vi "e.gate HighSpeedPort Query - Base.vi"(0 "e.gate Configuration in":T1 {"StartTime" format="%#.10f"; "dActTimeToSecondFactor" format="%#.10f"; "StartTimeToDayFactor" format="%#_10f"}, 1 "Command":i32, 2 "OffsetWrite":i32, 3 "LengthWrite":i32, 4 "DataWrite":string="\u0000\t\f\u0000\u0000\u0000\u0000", 5 "OffsetRead":i32, 6 "LengthRead":i32, 7 "error in (no error)":errorcluster, 9 "TCP LengthReadt":i32, 11 "Timeout (1000)":i32) -> (20 "e.gate Configuration out":T1 {"StartTime" format="%#.10f"; "dActTimeToSecondFactor" format="%#.10f"; "StartTimeToDayFactor" format="%#_10f"}, 23 "Data (out binary)":u8[](array[numeric]), 24 "data out (string)":string, 27 "error out":errorcluster)   [LabVIEW 2016]
doc: "This VI is used to build up the HighSpeedPort TCP/IP request frame and uses e.gate <B>HighSpeedPort Query</B> for data transfer."
uses:
  e.gate Configuration.ctl
  e.gate Channel Data.ctl
  e.gate Data Type.ctl
  e.gate Protocol Type.ctl
  e.gate Module  Data.ctl
  e.gateHSP_DLLhandle.ctl
panel:
  out "LengthWrite Buffer":string
  out "OffsetWrite Buffer":string
  out "Command Buffer":string
  out "DataWrite Buffer":string
  out "OffsetRead Buffer":string
  out "LengthRead Buffer":string
  out "LengthOfFrame Buffer":string
  out "Frame Buffer":string
  out "Frame Online":string
  out "LengthOfFrame":string
  out "LengthRead":string
  out "OffsetRead":string
  out "DataWrite":string
  out "LengthWrite":string
  out "OffsetWrite":string
  out "Command":string
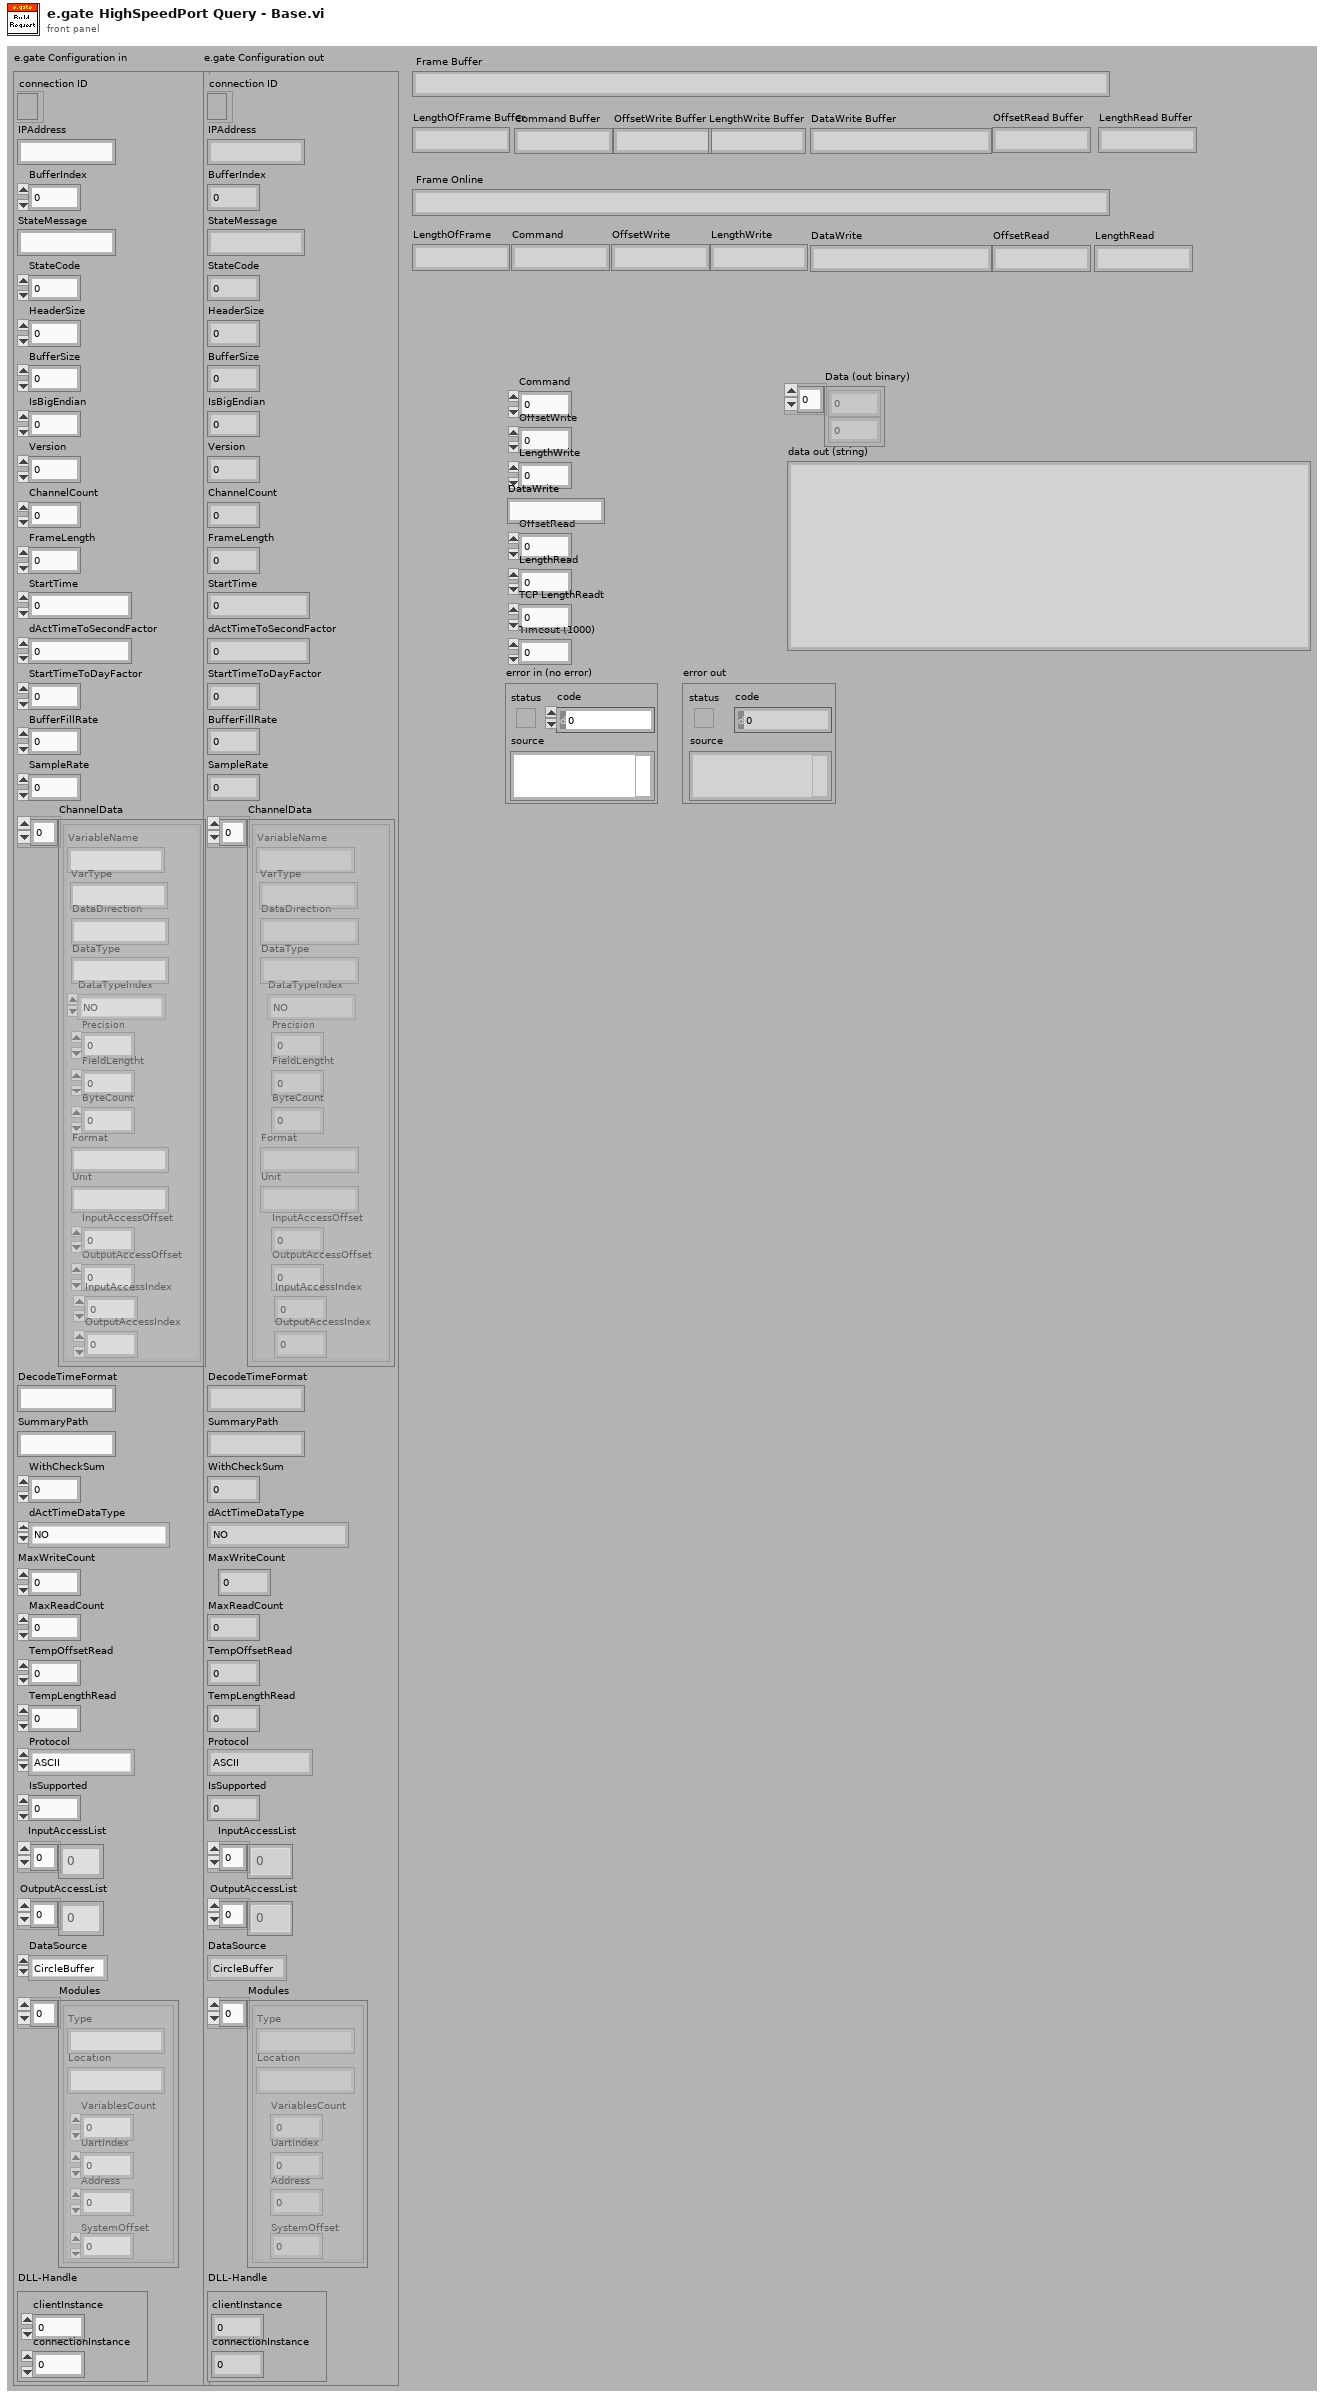
[diagram p1: front panel]
types:
  T1 = typedef "e.gate Configuration.ctl" = cluster{"connection ID":refnum<k5>, "IPAddress":string, "BufferIndex":i32, "StateMessage":string, "StateCode":i8, "HeaderSize":i32, "BufferSize":i32, "IsBigEndian":i32, "Version":i32, "ChannelCount":i32, "FrameLength":i32, "StartTime":dbl, "dActTimeToSecondFactor":dbl, "StartTimeToDayFactor":dbl, "BufferFillRate":dbl, "SampleRate":dbl, "ChannelData":T2[], "DecodeTimeFormat":string, "SummaryPath":string, "WithCheckSum":i32, "dActTimeDataType":T3, "MaxWriteCount":i32, "MaxReadCount":i32, "TempOffsetRead":i32, "TempLengthRead":i32, "Protocol":T4, "IsSupported":i32, "InputAccessList":i32[], "OutputAccessList":i32[], "DataSource":enum16{"CircleBuffer", "test.con Logger", "test.con Archive"}, "Modules":T5[], "DLL-Handle":T6}
  T2 = typedef "e.gate Channel Data.ctl" = cluster{"VariableName":string, "DataDirection":string, "DataType":string, "DataTypeIndex":T3, "Precision":i16, "FieldLengtht":i16, "ByteCount":i32, "Format":string, "Unit":string, "InputAccessOffset":i32, "OutputAccessOffset":i16, "InputAccessIndex":i16, "OutputAccessIndex":i16, "VarType":string}
  T3 = typedef "e.gate Data Type.ctl" = enum16{"NO", "BOOL", "SINT8", "USINT8", "SINT16", "USINT16", "SINT32", "USINT32", "FLOAT", "SET8", "SET16", "SET32", "DOUBLE", "SINT64", "USINT64", "SET64"}
  T4 = typedef "e.gate Protocol Type.ctl" = enum16{"ASCII", "HighspeedPort Online", "HighspeedPort Buffer", "eGateHighspeedPortDLL "}
  T5 = typedef "e.gate Module  Data.ctl" = cluster{"Type":string, "Location":string, "VariablesCount":i16, "UartIndex":i16, "Address":i16, "SystemOffset":i16}
  T6 = typedef "e.gateHSP_DLLhandle.ctl" = cluster{"clientInstance":i32, "connectionInstance":i32}
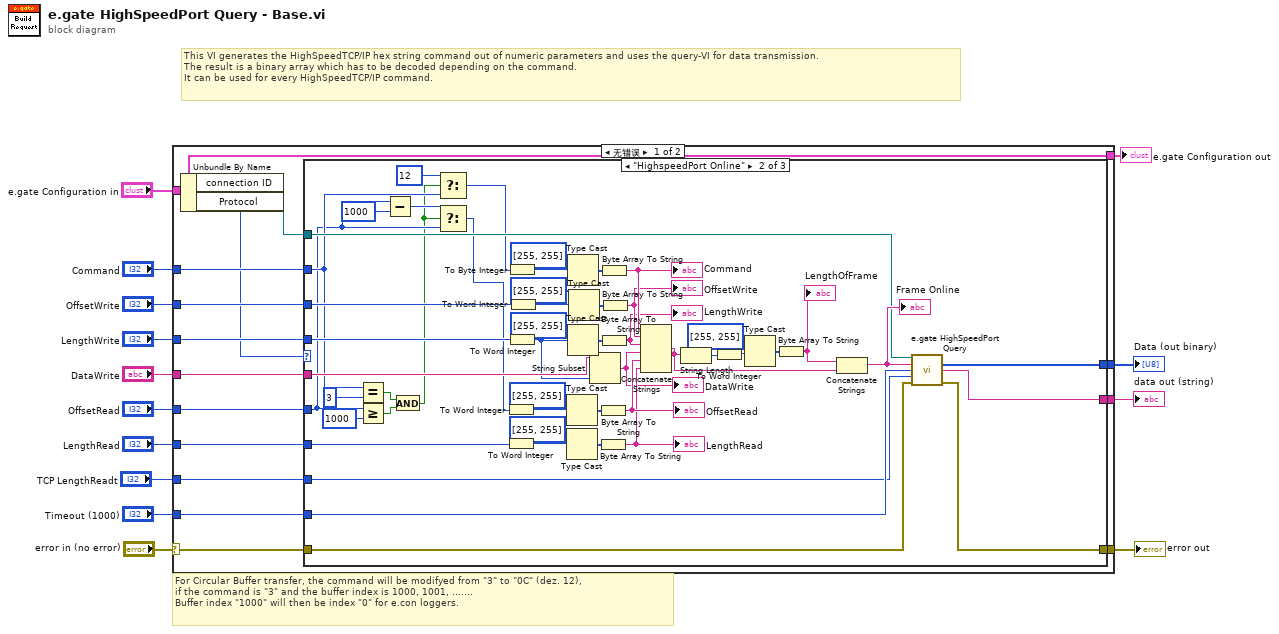
[diagram p0: block diagram]
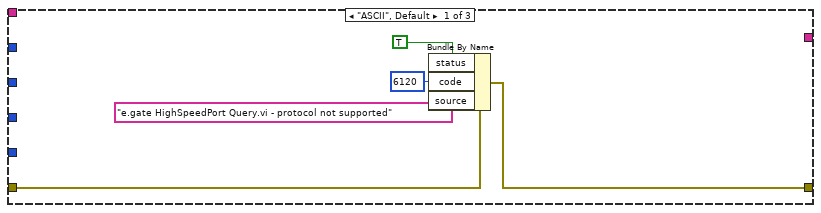
[diagram p2: hidden frame]
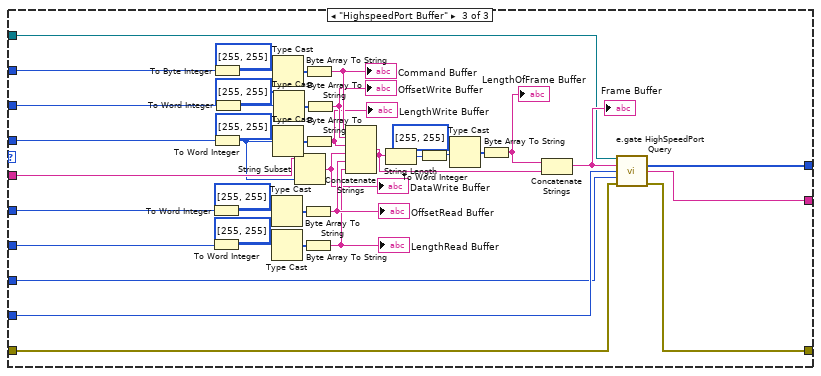
[diagram p3: hidden frame]
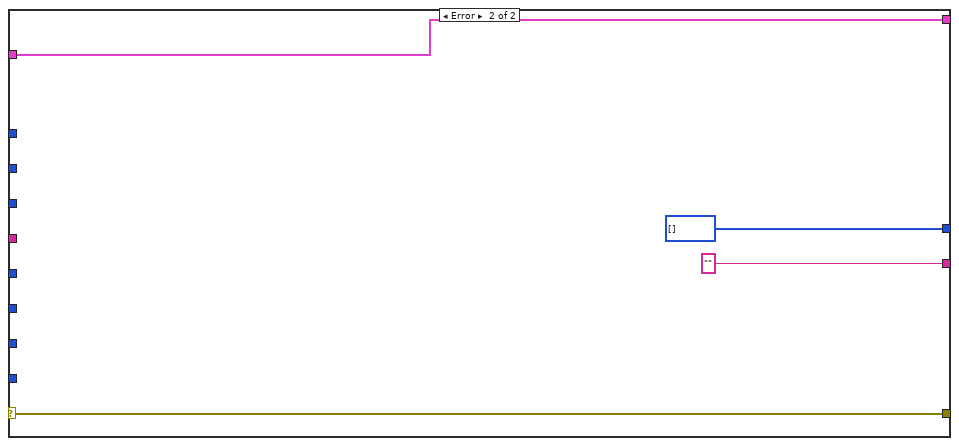
[diagram p4: hidden frame]
diagram:
  # "For Circular Buffer transfer, the command will be modifyed from \"3\" to \"0C\" (dez. 12),\nif the command is \"3\" and the buffer index is 1000, 1001, .......\nBuffer index \"1000\" will then be index \"0\" for e.con loggers."
  # "This VI generates the HighSpeedTCP/IP hex string command out of numeric parameters and uses the query-VI for data transmission.\nThe result is a binary array which has to be decoded depending on the command.\nIt can be used for every HighSpeedTCP/IP command."
  n1 = case shown="无错误" "error in (no error)" {
    selector: "error in (no error)" -> [w18 w130]
    tunnel: "Timeout (1000)" -> [w29 _]
    tunnel: "TCP LengthReadt" -> [w28 _]
    tunnel: "Command" -> [w20 _]
    tunnel: "OffsetRead" -> [w19 _]
    tunnel: "LengthRead" -> [w24 _]
    tunnel: "OffsetWrite" -> [w21 _]
    tunnel: "LengthWrite" -> [w25 _]
    tunnel: "DataWrite" -> [w23 _]
    tunnel: [w27 w130] -> w3
    tunnel: [w26 u8[] [] ("Data (out - binary)")] -> w7
    tunnel: [w22 "" ("data out (string)")] -> w5
    tunnel: "e.gate Configuration in" -> [w16 w127]
    tunnel: [w16 w127] -> w1
    frame No Error {
      n2 = Unbundle By Name(w16) -> ("connection ID"=w15:refnum<k5>, "Protocol"=w17:T4)
      n3 = case shown="\"HighspeedPort Online\"" w17 {
        tunnel: w29 -> [_ w84 w125]
        tunnel: w28 -> [_ w83 w124]
        tunnel: w15 -> [_ w82 w123]
        tunnel: [w34 w81 w122] -> w27
        tunnel: [_ w80 w121] -> w26
        tunnel: w25 -> [_ w69 w110]
        tunnel: w24 -> [_ w62 w103]
        tunnel: w23 -> [_ w54 w95]
        tunnel: [_ w51 w92] -> w22
        tunnel: w21 -> [_ w47 w89]
        tunnel: w20 -> [_ w42 w86]
        tunnel: w19 -> [_ w39 w87]
        tunnel: w18 -> [w33 w35 w88]
        frame "ASCII", Default {
          n4 = Bundle By Name(cluster=w33, "status"=TRUE, "code"=6120, "source"="e.gate HighSpeedPort Query.vi - protocol not supported") -> (w34:errorcluster)
        }
        frame "HighspeedPort Online" {
          n5 = Equal?(x=w42, y=3) -> (x = y?=w45:bool)
          n6 = Greater Or Equal?(x=w39, y=1000) -> (x >= y?=w46:bool)
          n7 = Subtract(x=w39, y=1000) -> (x-y=w40:i32)
          n8 = And(x=w45, y=w46) -> (x .and. y?=w37:bool)
          n9 = Select(t=12 ("Command"), s=w37, f=w42) -> (s? t:f=w41:i32)
          n10 = Select(t=w40, s=w37, f=w39) -> (s? t:f=w36:i32)
          n11 = To Word Integer(number=w36) -> (16bit integer=w66:i16)
          n12 = To Word Integer(number=w62) -> (16bit integer=w63:i16)
          n13 = To Byte Integer(number=w41) -> (8bit integer=w77:i8)
          n14 = To Word Integer(number=w69) -> (16bit integer=w49:i16)
          n15 = To Word Integer(number=w47) -> (16bit integer=w73:i16)
          n16 = Type Cast(type=u8[] [255, 255] ("Vorzeichenloses Byte-Array"), x=w66) -> (*(type *) &x=w67:u8[])
          n17 = Type Cast(type=u8[] [255, 255] ("Vorzeichenloses Byte-Array"), x=w63) -> (*(type *) &x=w64:u8[])
          n18 = Type Cast(type=u8[] [255, 255] ("Vorzeichenloses Byte-Array"), x=w77) -> (*(type *) &x=w78:u8[])
          n19 = Type Cast(type=u8[] [255, 255] ("Vorzeichenloses Byte-Array"), x=w49) -> (*(type *) &x=w70:u8[])
          n20 = Type Cast(type=u8[] [255, 255] ("Vorzeichenloses Byte-Array"), x=w73) -> (*(type *) &x=w74:u8[])
          n21 = String Subset(string=w54, length (rest)=w49) -> (substring=w53:string)  [unwired: 1 out]
          "DataWrite" <- w53
          n22 = Byte Array To String(unsigned byte array=w67) -> (string=w61:string)
          "OffsetRead" <- w61
          n23 = Byte Array To String(unsigned byte array=w64) -> (string=w60:string)
          "LengthRead" <- w60
          n24 = Byte Array To String(unsigned byte array=w78) -> (string=w76:string)
          "Command" <- w76
          n25 = Byte Array To String(unsigned byte array=w70) -> (string=w52:string)
          "LengthWrite" <- w52
          n26 = Byte Array To String(unsigned byte array=w74) -> (string=w72:string)
          "OffsetWrite" <- w72
          n27 = Concatenate Strings(w76, w72, w52, w53, w61, w60) -> (w55:string)
          n28 = String Length(string=w55) -> (length=w50:i32)
          n29 = To Word Integer(number=w50) -> (16bit integer=w59:i16)
          n30 = Type Cast(type=u8[] [255, 255] ("Vorzeichenloses Byte-Array"), x=w59) -> (*(type *) &x=w58:u8[])
          n31 = Byte Array To String(unsigned byte array=w58) -> (string=w56:string)
          "LengthOfFrame" <- w56
          n32 = Concatenate Strings(w56, w55) -> (w85:string)
          "Frame Online" <- w85
          n33 = call "e.gate HighSpeedPort Query.vi"("TCP-Connection (Refnum in)"=w82, "Command (In)"=w85, "Timeout"=w84, "TCP LengthRead"=w83, "error in (no error)"=w35) -> ("Data (out - binary)"=w80:u8[], "data out (string)"=w51:string, "error out"=w81:errorcluster)  [unwired: 8 out]
        }
        frame "HighspeedPort Buffer" {
          n34 = To Word Integer(number=w87) -> (16bit integer=w107:i16)
          n35 = To Word Integer(number=w103) -> (16bit integer=w104:i16)
          n36 = To Byte Integer(number=w86) -> (8bit integer=w118:i8)
          n37 = To Word Integer(number=w110) -> (16bit integer=w90:i16)
          n38 = To Word Integer(number=w89) -> (16bit integer=w114:i16)
          n39 = Type Cast(type=u8[] [255, 255] ("Vorzeichenloses Byte-Array"), x=w107) -> (*(type *) &x=w108:u8[])
          n40 = Type Cast(type=u8[] [255, 255] ("Vorzeichenloses Byte-Array"), x=w104) -> (*(type *) &x=w105:u8[])
          n41 = Type Cast(type=u8[] [255, 255] ("Vorzeichenloses Byte-Array"), x=w118) -> (*(type *) &x=w119:u8[])
          n42 = Type Cast(type=u8[] [255, 255] ("Vorzeichenloses Byte-Array"), x=w90) -> (*(type *) &x=w111:u8[])
          n43 = Type Cast(type=u8[] [255, 255] ("Vorzeichenloses Byte-Array"), x=w114) -> (*(type *) &x=w115:u8[])
          n44 = String Subset(string=w95, length (rest)=w90) -> (substring=w94:string)  [unwired: 1 out]
          "DataWrite Buffer" <- w94
          n45 = Byte Array To String(unsigned byte array=w108) -> (string=w102:string)
          "OffsetRead Buffer" <- w102
          n46 = Byte Array To String(unsigned byte array=w105) -> (string=w101:string)
          "LengthRead Buffer" <- w101
          n47 = Byte Array To String(unsigned byte array=w119) -> (string=w117:string)
          "Command Buffer" <- w117
          n48 = Byte Array To String(unsigned byte array=w111) -> (string=w93:string)
          "LengthWrite Buffer" <- w93
          n49 = Byte Array To String(unsigned byte array=w115) -> (string=w113:string)
          "OffsetWrite Buffer" <- w113
          n50 = Concatenate Strings(w117, w113, w93, w94, w102, w101) -> (w96:string)
          n51 = String Length(string=w96) -> (length=w91:i32)
          n52 = To Word Integer(number=w91) -> (16bit integer=w100:i16)
          n53 = Type Cast(type=u8[] [255, 255] ("Vorzeichenloses Byte-Array"), x=w100) -> (*(type *) &x=w99:u8[])
          n54 = Byte Array To String(unsigned byte array=w99) -> (string=w97:string)
          "LengthOfFrame Buffer" <- w97
          n55 = Concatenate Strings(w97, w96) -> (w126:string)
          "Frame Buffer" <- w126
          n56 = call "e.gate HighSpeedPort Query.vi"("TCP-Connection (Refnum in)"=w123, "Command (In)"=w126, "Timeout"=w125, "TCP LengthRead"=w124, "error in (no error)"=w88) -> ("Data (out - binary)"=w121:u8[], "data out (string)"=w92:string, "error out"=w122:errorcluster)  [unwired: 8 out]
        }
      }
    }
    frame Error {
    }
  }
  "Data (out binary)" <- w7
  "data out (string)" <- w5
  "error out" <- w3
  "e.gate Configuration out" <- w1
